vi "PIM Execute Measurement.vi"(0 "TestSetDef":T3={"General"={"ID"=0, "Model"="", "Dual Port?"=FALSE, "Options"="", "Options"={"E"=FALSE, "K"=FALSE, "H"=FALSE, "W"=FALSE, "F"=FALSE}, "Cal File"=path ""}, "Receiver"={"Fstart, MHz"=0.0, "Fstop MHz"=0.0, "Fstep MHz"=0.0, "IF, MHz"=0.0}, "RX Band"={"Fstart, MHz"=0.0, "Fstop MHz"=0.0}, "TX 1"={"Fstart, MHz"=0.0, "Fstop MHz"=0.0, "Pmax, dBm"=0.0, "Pstep, dB"=0.0}, "TX 2"={"Fstart, MHz"=0.0, "Fstop MHz"=0.0, "Pmax, dBm"=0.0, "Pstep, dB"=0.0}, "Low-side?"=TRUE}, 5 "PIM Test Parameters":T4={"Stimulus"={"C1 Pwr dBm"=0.0, "C2 Pwr dBm"=0.0, "Power Units"=enum."dBm", "Meas Type"=enum."Time", "C1 Freq MHz"=0.0, "C2 Freq MHz"=0.0, "Swept Freq Step"=0}, "Measure"={"IM Order"=0, "Direction"=0, "Averaging"=1, "ALC ON?"=TRUE, "Peak Hold?"=TRUE, "Peak last N"=1, "Ref Level dBm"=-100.0, "Ref Units"=enum."dBm", "Num Samples"=1, "Sample units"=enum."Sample(s)", "Update Rate (s)"=0.0, "DUT PORT"=enum."Port 1", "Percent (%)"=100}, "Display"={"Power Scale"={"yRange_min"=0, "yRange_max"=0}, "xRange_span"=5}} {"Stimulus"."Swept Freq Step" items=[".2", ".4", "1.0", "2.0"]; "Measure"."Averaging" items=["None", "Minimum", "Normal", "High", "Maximum"]; "Measure"."Direction" items=["Reverse", "Forward", "Auxiliary"]; "Measure"."IM Order" items=["3rd", "5th", "7th", "9th", "11th", "13th", "15th", "17th", "19th", "21st", "23rd", "25th", "27th", "29th", "31st", "33rd"]}, 7 "Freq Display Ref":refnum<vi>, 9 "Restart Meas?":bool, 11 "error in (no error)":errorcluster, 12 "Driver Ref":T1) -> (1 "Actual Peak Samples":i32, 2 "Discarded?":bool, 3 "Peak Value":dbl, 4 "Meas Results":T2 {"IMPower_dBc(s)" format="%.2f"; "TxFreqs" format="%.2f"; "IMFreq(s)" format="%.2f"; "IMPower(s)" format="%.2f"; "TxPower" format="%.2f"}, 6 "Passed?":bool, 8 "Done?":bool, 10 "% Complete":dbl, 13 "% Passed":dbl, 14 "dup driver ref":T1, 15 "error out":errorcluster)   [LabVIEW 2011]
uses:
  TypeDefs/PIM Test Parameters.ctl
  TypeDefs/PIM Stimulus Parameters.ctl
  SI.LIB/PIM.LIB/HW IO/PIM Sweep Step Size.ctl
  TypeDefs/PIM Measurement Parameters.ctl
  SI.LIB/PIM.LIB/HW IO/IMOrder.ctl
  SI.LIB/PIM.LIB/HW IO/MeasMode.ctl
  SI.LIB/PIM.LIB/HW IO/HW Averaging.ctl
  TypeDefs/PIM Meas Units.ctl
  SI.LIB/PIM.LIB/HW IO/DUTport.ctl
  TypeDefs/PIM Display Parameters.ctl
  SI.LIB/PIM.LIB/HW IO/Test Set Definition.ctl
  drivers/PIM/PIM Driver Ref.ctl
  drivers/PIM/PIM Results.ctl
  drivers/PIM/PIM Command.ctl
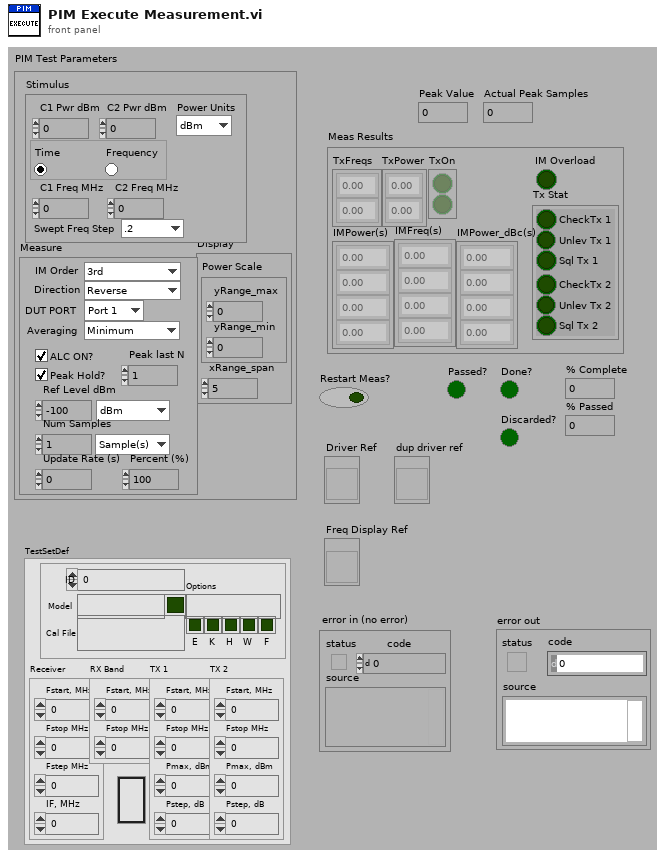
[diagram p1: front panel]
types:
  T1 = typedef "PIM Driver Ref.ctl" = refnum<vi>
  T2 = typedef "PIM Results.ctl" = cluster{"TxFreqs":dbl[], "TxPower":dbl[], "TxOn":bool[], "IMPower(s)":dbl[], "IMFreq(s)":dbl[], "Tx Stat":cluster{"CheckTx 1":bool, "Unlev Tx 1":bool, "Sql Tx 1":bool, "CheckTx 2":bool, "Unlev Tx 2":bool, "Sql Tx 2":bool}, "IM Overload":bool, "IMPower_dBc(s)":dbl[]}
  T3 = typedef "Test Set Definition.ctl" = cluster{"General":cluster{"ID":u32, "Model":string, "Dual Port?":bool, "Options":string, "Options":cluster{"E":bool, "K":bool, "H":bool, "W":bool, "F":bool}, "Cal File":path}, "Receiver":cluster{"Fstart, MHz":dbl, "Fstop MHz":dbl, "Fstep MHz":dbl, "IF, MHz":dbl}, "RX Band":cluster{"Fstart, MHz":dbl, "Fstop MHz":dbl}, "TX 1":cluster{"Fstart, MHz":dbl, "Fstop MHz":dbl, "Pmax, dBm":dbl, "Pstep, dB":dbl}, "TX 2":cluster{"Fstart, MHz":dbl, "Fstop MHz":dbl, "Pmax, dBm":dbl, "Pstep, dB":dbl}, "Low-side?":bool}
  T4 = typedef "PIM Test Parameters.ctl" = cluster{"Stimulus":T5, "Measure":T7, "Display":T13}
  T5 = typedef "PIM Stimulus Parameters.ctl" = cluster{"C1 Pwr dBm":dbl, "C2 Pwr dBm":dbl, "Power Units":enum16{"dBm", "Watts"}, "Meas Type":enum32{"Time", "Frequency"}, "C1 Freq MHz":dbl, "C2 Freq MHz":dbl, "Swept Freq Step":T6}
  T6 = typedef "PIM Sweep Step Size.ctl" = u16
  T7 = typedef "PIM Measurement Parameters.ctl" = cluster{"IM Order":T8, "Direction":T9, "Averaging":T10, "ALC ON?":bool, "Peak Hold?":bool, "Peak last N":u32, "Ref Level dBm":dbl, "Ref Units":enum16{"dBm", "dBc"}, "Num Samples":u32, "Sample units":T11, "Update Rate (s)":dbl, "DUT PORT":T12, "Percent (%)":u8}
  T8 = typedef "IMOrder.ctl" = u8
  T9 = typedef "MeasMode.ctl" = u16
  T10 = typedef "HW Averaging.ctl" = u16
  T11 = typedef "PIM Meas Units.ctl" = enum16{"Sample(s)", "Second(s)", "Sweep(s)"}
  T12 = typedef "DUTport.ctl" = enum16{"Port 1", "Port 2"}
  T13 = typedef "PIM Display Parameters.ctl" = cluster{"Power Scale":cluster{"yRange_min":i32, "yRange_max":i32}, "xRange_span":u32}
  T14 = typedef "PIM Command.ctl" = enum16{"LOAD", "KEEP ALIVE", "VALIDATE", "INITIALIZE", "PRESET", "GET CALIBRATION", "SET STIMULUS", "TOGGLE TX POWER", "SET TX ON", "SET TX OFF", "MEASURE", "UNLOAD"}
  T15 = typedef "PIM Stimulus.ctl" = cluster{"Carrier Frequencies":cluster{"C1 Freq, MHz":dbl, "C2 Freq, MHz":dbl}, "Carrier Powers":cluster{"C1 Power,dBm":dbl, "C2 Power, dBm":dbl}, "Measurement Parameters":T16, "Measurement Setup":cluster{"Meas Type":enum32{"Time", "Frequency"}, "TXStep":T6}}
  T16 = typedef "PIM Cmd Params.ctl" = cluster{"IM Order":T8, "Averaging":T10, "Direction":T9, "Enable ALC?":bool, "Enable SingleIM?":bool, "Display Units":T17, "VA Hold?":bool, "DUT PORT":T12}
  T17 = typedef "display_unit_format.ctl" = enum16{"dBm", "dBc"}
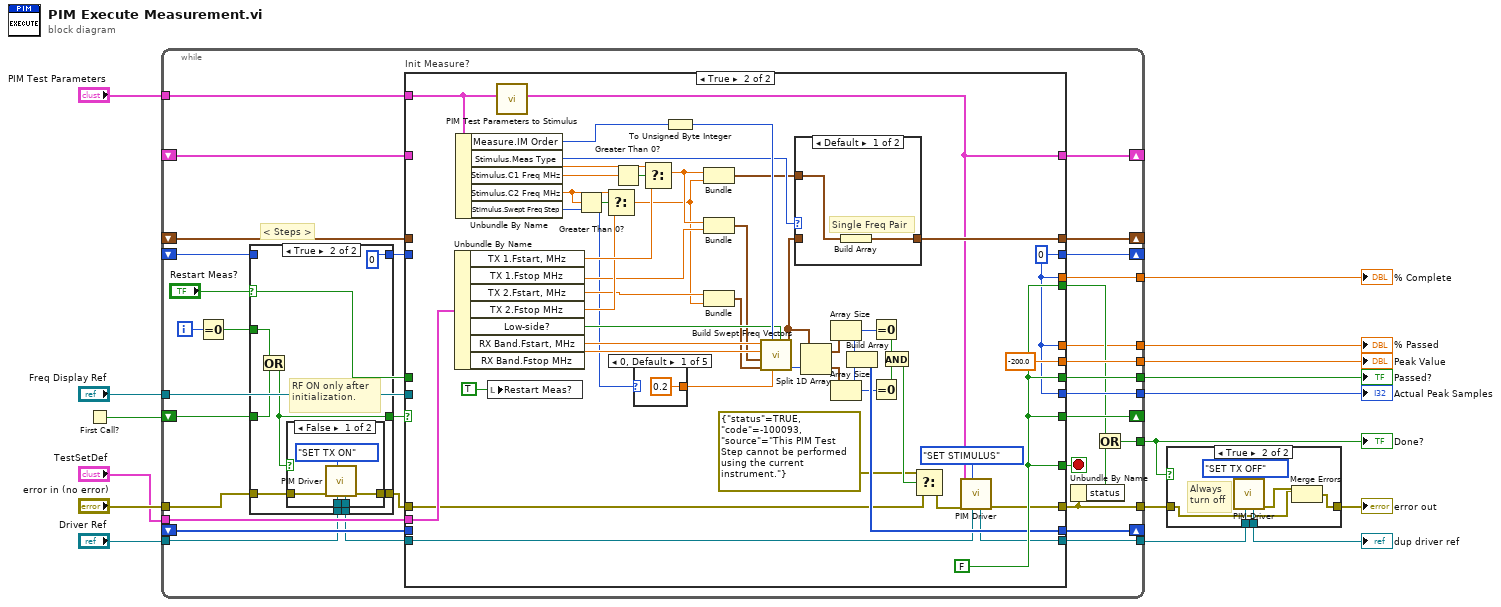
[diagram p0: block diagram]
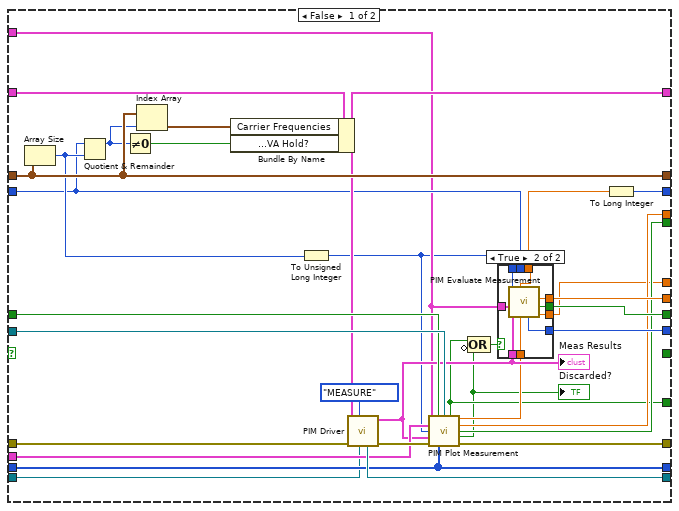
[diagram p5: hidden frame]
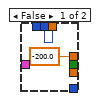
[diagram p6: hidden frame]
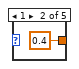
[diagram p7: hidden frame]
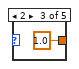
[diagram p8: hidden frame]
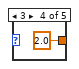
[diagram p9: hidden frame]
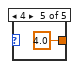
[diagram p10: hidden frame]
diagram:
  n1 = First Call?() -> (First Call?: T/F=w3:bool)
  n2 = while {
    tunnel: "PIM Test Parameters" -> [w49]
    tunnel: "TestSetDef" -> [w48]
    shift-right: [w47] -> _
    shift-left: _ -> [w46]
    shift-right: [w44] -> _
    shift-left: _ -> [w35]
    tunnel: [w43] -> w15
    tunnel: [w24] -> w6
    tunnel: "error in (no error)" -> [w33]
    tunnel: "Driver Ref" -> [w31]
    tunnel: [w27] -> w10
    tunnel: [w42] -> w8
    tunnel: [w41] -> w12
    tunnel: [w40] -> w11
    shift-right: [w39] -> _
    shift-left: w3 -> [w23]
    shift-right: [w38] -> _
    shift-left: _ -> [w37]
    tunnel: "Freq Display Ref" -> [w36]
    tunnel: [w28] -> w2
    shift-right: [w21] -> _
    shift-left: _ -> [w20]
    tunnel: [w19] -> w1
    i -> [w18]
    stop <- w45 stop-if-true
    # "< Steps >"
    n3 = Equal To 0?(x=w18) -> (x = 0?=w17:bool)
    n4 = case shown="True" "Restart Meas?" {
      tunnel: w33 -> [w52 w61]
      tunnel: [w52 w60] -> w32
      tunnel: w31 -> [w53 w59]
      tunnel: [w53 w58] -> w30
      tunnel: w35 -> [w51 _]
      tunnel: [w51 0 ("Updated Count")] -> w34
      tunnel: w23 -> [w50 w56]
      tunnel: [w50 w54] -> w22
      tunnel: w17 -> [_ w55]
      frame False {
        # "Carriers should be\non already (unless\na HW error occurred)"
      }
      frame True {
        # "RF ON only after initialization."
        n5 = Or(x=w55, y=w56) -> (x .or. y?=w54:bool)
        n6 = case shown="False" w54 {
          tunnel: w61 -> [w66 w67]
          tunnel: [w65 w67] -> w60
          tunnel: w59 -> [w63 w68]
          tunnel: [w62 w68] -> w58
          frame False {
            n7 = call "PIM Driver.vi"("Driver Ref (null)"=w63, "PIM Command"=PIM_Command."SET TX ON", "error in (no error)"=w66) -> ("error out"=w65:errorcluster, "duplicate driver ref"=w62:T1)  [unwired: 2 in, 5 out]
          }
          frame True {
          }
        }
      }
    }
    n8 = case "Init Measure?" shown="True" w22 {
      tunnel: w49 -> [w76 w125]
      tunnel: w48 -> [w90 w157]
      tunnel: [w101 w142] -> w47
      tunnel: w46 -> [w101 _]
      tunnel: [w72 w136] -> w45
      tunnel: [w85 w112] -> w44
      tunnel: w34 -> [w77 _]
      tunnel: [w74 w112] -> w43
      tunnel: [w73 w136] -> w26
      tunnel: w32 -> [w89 w126]
      tunnel: w30 -> [w88 w116]
      tunnel: [w93 w117] -> w27
      tunnel: [w98 w115] -> w42
      tunnel: [w97 w136] -> w41
      tunnel: [w96 -200.0 ("Peak Value")] -> w40
      tunnel: [_ w136] -> w39
      tunnel: [w91 w135] -> w38
      tunnel: w37 -> [w91 _]
      tunnel: w36 -> [w92 _]
      tunnel: "Restart Meas?" -> [w87 _]
      tunnel: [w86 w112] -> w28
      tunnel: [w81 w119] -> w21
      tunnel: w20 -> [w82 _]
      tunnel: [w69 w112] -> w19
      frame False {
        n9 = Array Size(array=w101) -> (size(s)=w79:i32)
        n10 = Quotient & Remainder(x=w77, y=w79) -> (x-y*floor(x/y)=w84:i32)  [unwired: 1 out]
        n11 = Not Equal To 0?(x=w84) -> (x != 0?=w83:bool)
        n12 = Index Array(array=w101, index=w84) -> (element=w99:cluster{"F(C1)":dbl, "F(C2)":dbl})
        n13 = Bundle By Name(cluster=w82, "Carrier Frequencies"=w99, "Measurement Parameters.VA Hold?"=w83) -> (w81:T15)
        n14 = To Unsigned Long Integer(number=w79) -> (unsigned 32bit integer=w75:u32)
        n15 = call "PIM Driver.vi"("Driver Ref (null)"=w88, "PIM Command"=PIM_Command."MEASURE", "error in (no error)"=w89, "Stimulus"=w81) -> ("error out"=w94:errorcluster, "Measurement Results"=w80:T2, "duplicate driver ref"=w98:T1)  [unwired: 1 in, 4 out]
        "Meas Results" <- w80
        n16 = call "PIM Plot Measurement.vi"("PIM Test Parameters"=w76, "Reset Plot?"=w87, "Freq Display Ref"=w92, "TestSetDef"=w90, "Steps Per Sample"=w75, "Measurement Results"=w80, "error in (no error)"=w94, "Sweep Sizes"=w91) -> ("Point Plotted?"=w72:bool, "Current Count"=w78:dbl, "Percent Complete"=w74:dbl, "Done?"=w73:bool, "Discarded?"=w71:bool, "error out"=w93:errorcluster)  [unwired: 2 out]
        "Discarded?" <- w71
        n17 = Compound Arithmetic op=OR(w72, invert w71) -> (w70:bool)
        n18 = case shown="True" w70 {
          tunnel: [_ w111] -> w97
          tunnel: [-200.0 ("% Complete") w110] -> w96
          tunnel: [w103 w105] -> w95
          tunnel: w75 -> [_ w109]
          tunnel: w76 -> [_ w108]
          tunnel: w80 -> [_ w107]
          tunnel: [_ w106] -> w86
          tunnel: w78 -> [_ w105]
          tunnel: w77 -> [w103 _]
          tunnel: [_ w104] -> w69
          frame False {
          }
          frame True {
            n19 = call "PIM Evaluate Measurement.vi"("Current Count"=w105, "Measurement Results"=w107, "PIM Test Parameters"=w108, "Steps per sample"=w109) -> ("% Passed"=w104:dbl, "Passed Limits?"=w111:bool, "Peak Value"=w110:dbl, "Actual Peak Samples"=w106:i32)  [unwired: 1 in, 3 out]
          }
        }
        n20 = To Long Integer(number=w95) -> (32bit integer=w85:i32)
      }
      frame True {
        w136 = FALSE
        w112 = 0
        n21 = Unbundle By Name(w157) -> ("TX 1.Fstart, MHz"=w149:dbl, "TX 1.Fstop MHz"=w147:dbl, "TX 2.Fstart, MHz"=w146:dbl, "TX 2.Fstop MHz"=w148:dbl, "Low-side?"=w152:bool, "RX Band.Fstart, MHz"=w156:dbl, "RX Band.Fstop MHz"=w155:dbl)
        n22 = Unbundle By Name(w125) -> ("Measure.IM Order"=w154:T8, "Stimulus.Meas Type"=w143:enum32{"Time", "Frequency"}, "Stimulus.C1 Freq MHz"=w151:dbl, "Stimulus.C2 Freq MHz"=w150:dbl, "Stimulus.Swept Freq Step"=w114:T6)
        n23 = local write "Restart Meas?"(TRUE ("Restart Meas?")) -> ()
        n24 = call "PIM Test Parameters to Stimulus.vi"("PIM Test Parameters"=w125) -> ("PIM Measurement Stimulus"=w119:T15)  [unwired: 10 out]
        n25 = Greater Than 0?(x=w150) -> (x > 0?=w123:bool)
        n26 = Select(t=w150, s=w123, f=w148) -> (s? t:f=w121:dbl)
        n27 = Greater Than 0?(x=w151) -> (x > 0?=w124:bool)
        n28 = case shown="0, Default" w114 {
          tunnel: [0.2 ("Freq. Increment MHz") 0.4 ("Freq. Increment MHz") 1.0 ("Freq. Increment MHz") 2.0 ("Freq. Increment MHz") 4.0 ("Freq. Increment MHz")] -> w113
          frame 0, Default {
          }
          frame 1 {
          }
          frame 2 {
          }
          frame 3 {
          }
          frame 4 {
          }
        }
        n29 = Select(t=w151, s=w124, f=w149) -> (s? t:f=w122:dbl)
        n30 = To Unsigned Byte Integer(number=w154) -> (unsigned 8bit integer=w153:T8)
        n31 = Bundle("Fstart, MHz"=w122, "Fstop MHz"=w121) -> (w134:cluster{"Fstart, MHz":dbl, "Fstop MHz":dbl})  [unwired: 1 out]
        n32 = Bundle("Fstart, MHz"=w122, "Fstop MHz"=w147) -> (w145:cluster{"Fstart, MHz":dbl, "Fstop MHz":dbl})  [unwired: 1 out]
        n33 = Bundle("Fstart, MHz"=w146, "Fstop MHz"=w121) -> (w144:cluster{"Fstart, MHz":dbl, "Fstop MHz":dbl})  [unwired: 1 out]
        n34 = call "Build Swept Freq Vectors.vi"("Low or High (T=Low)"=w152, "Freq. Increment MHz"=w113, "Base Order (0)"=w153, "Carrier 2"=w144, "Carrier 1"=w145, "Rx High Freq"=w155, "Rx Low Freq"=w156) -> ("F2>F1 Changeover Index"=w140:i32, "Freq Sweep"=w139:cluster{"F(C1)":dbl, "F(C2)":dbl}[])  [unwired: 3 out]
        n35 = case shown="Default" w143 {
          tunnel: w139 -> [_ w165]
          tunnel: [w164 w165] -> w142
          tunnel: w134 -> [w163 _]
          frame Default {
            # "Single Freq Pair"
            n36 = Build Array(w163) -> (w164:cluster{"Fstart, MHz":dbl, "Fstop MHz":dbl}[])
          }
          frame "Frequency" {
          }
        }
        n37 = Split 1D Array(array=w139, index=w140) -> (first subarray=w138:cluster{"F(C1)":dbl, "F(C2)":dbl}[], second subarray=w137:cluster{"F(C1)":dbl, "F(C2)":dbl}[])
        n38 = Array Size(array=w138) -> (size(s)=w131:i32)
        n39 = Array Size(array=w137) -> (size(s)=w132:i32)
        n40 = Build Array(w131, w132) -> (w135:i32[])
        n41 = Equal To 0?(x=w131) -> (x = 0?=w130:bool)
        n42 = Equal To 0?(x=w132) -> (x = 0?=w129:bool)
        n43 = And(x=w130, y=w129) -> (x .and. y?=w128:bool)
        n44 = Select(t=errorcluster {"status"=TRUE, "code"=-100093, "source"="This PIM Test Step cannot be performed using the current instrument."} ("error out"), s=w128, f=w126) -> (s? t:f=w118:errorcluster)
        n45 = call "PIM Driver.vi"("Driver Ref (null)"=w116, "PIM Command"=PIM_Command."SET STIMULUS", "error in (no error)"=w118, "Stimulus"=w119) -> ("error out"=w117:errorcluster, "duplicate driver ref"=w115:T1)  [unwired: 1 in, 5 out]
      }
    }
    n46 = Unbundle By Name(w27) -> ("status"=w25:bool)
    n47 = Or(x=w26, y=w25) -> (x .or. y?=w24:bool)
  }
  "% Complete" <- w15
  "Done?" <- w6
  "Passed?" <- w12
  "Peak Value" <- w11
  "Actual Peak Samples" <- w2
  "% Passed" <- w1
  n48 = case shown="True" w6 {
    tunnel: w10 -> [w166 w168]
    tunnel: [w167 w172] -> w9
    tunnel: w8 -> [w167 w171]
    tunnel: [w166 w170] -> w7
    frame False {
    }
    frame True {
      # "Always\nturn off"
      n49 = call "PIM Driver.vi"("Driver Ref (null)"=w171, "PIM Command"=PIM_Command."SET TX OFF") -> ("error out"=w169:errorcluster, "duplicate driver ref"=w172:T1)  [unwired: 3 in, 5 out]
      n50 = Merge Errors(w168, w169) -> (w170:errorcluster)
    }
  }
  "error out" <- w7
  "dup driver ref" <- w9
